vi "FPGA_DAC_buses_v2.vi"() -> ()   [LabVIEW 2013]
uses:
  <vilib>/rvi/Emulation/niFpgaSctlEmulationGetInTimedLoop.vi
  <vilib>/rvi/Memory/Memory_Emulation/niFpgaMemoryEmulationReadFromVariant.vi
  <vilib>/rvi/Memory/Memory_Emulation/niFpgaMemoryEmulationWriteToVariant.vi
  <vilib>/rvi/DataTransferAndStorage/Container/Common/niFpgaContainerGetUniqueNameForEmu.vi
  <vilib>/rvi/FIFO/Fifo_Resource/nirvififoEmulationSetSize.vi
  <vilib>/rvi/errors/niFpgaSetErrorForExecOnDevCompSimple.vi
  <vilib>/rvi/eio/common/nirviEmuReportErrorAndStop.vi
  <vilib>/rvi/Emulation/niFpgaSctlEmulationFifoFullMgr.vi
  <vilib>/rvi/Emulation/niFpgaSctlEmulationResourceMgr.vi
  <vilib>/rvi/Memory/Memory_Emulation/nirvimemoryFastEmulation.vi
  <vilib>/rvi/Memory/Memory_Emulation/nirvimemoryEmulation.vi
  <vilib>/rvi/DataTransferAndStorage/Container/XNode/niFpgaContainer.xnode
  <vilib>/rvi/FIFO/Fifo_Resource/nirvififoEmulationWrite.vi
  <vilib>/rvi/FIFO/Fifo_Resource/nirvififoEmulationRead.vi
panel:
  in  "wait(us)":u16
  in  "start movement":bool
  in  "buses to use":bool[](array[boolean])=[FALSE, FALSE, FALSE, FALSE, FALSE, FALSE, FALSE, FALSE]
  in  "stop moving bus":bool
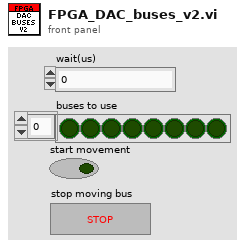
[diagram p1: front panel]
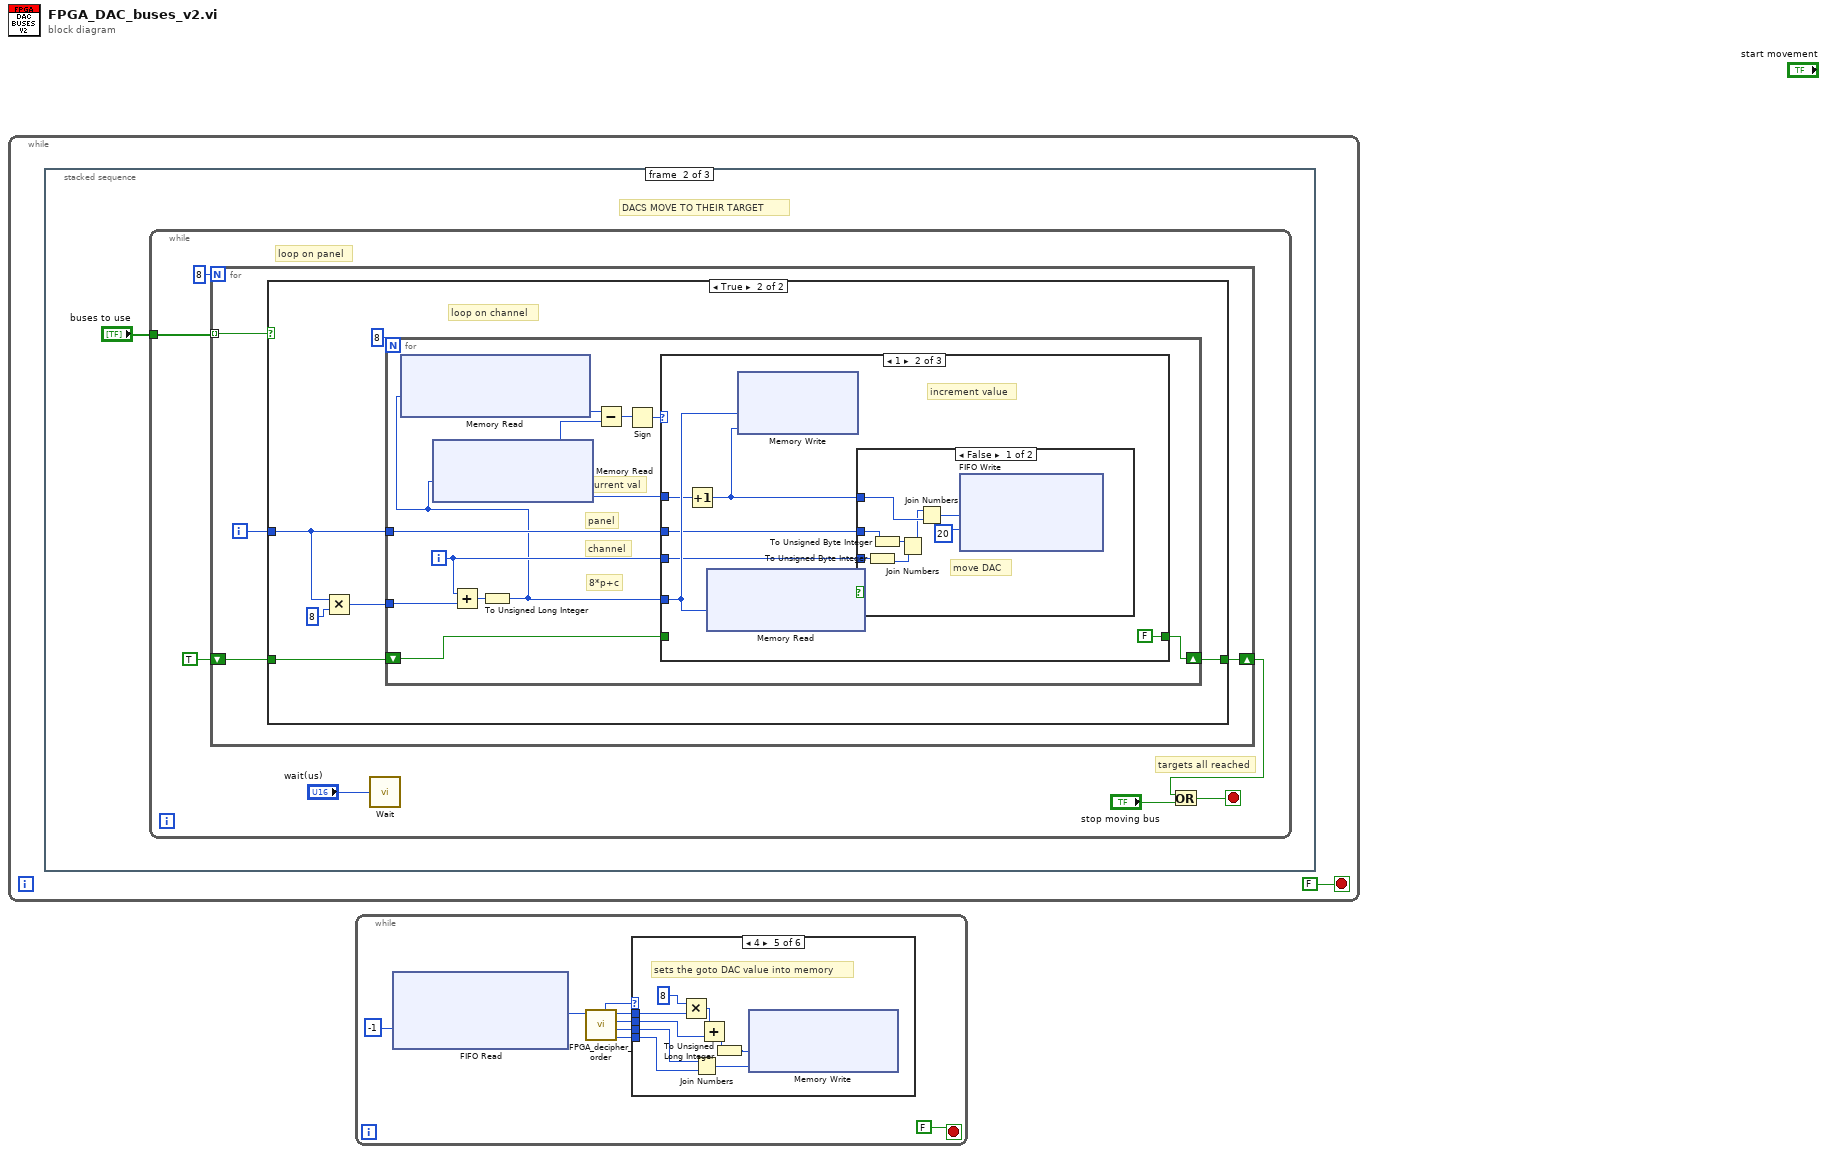
[diagram p0: block diagram]
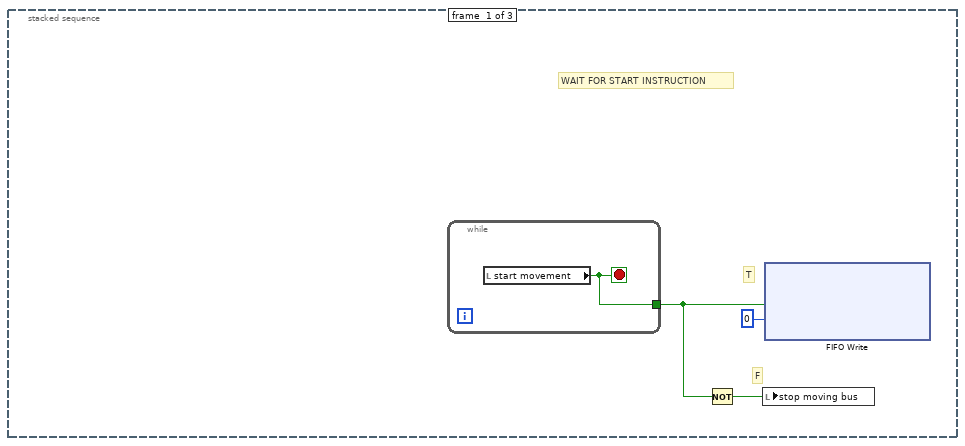
[diagram p2: hidden frame]
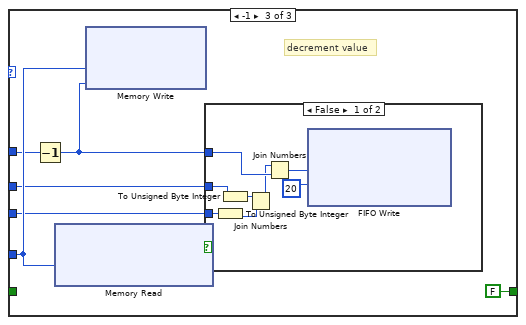
[diagram p6: hidden frame]
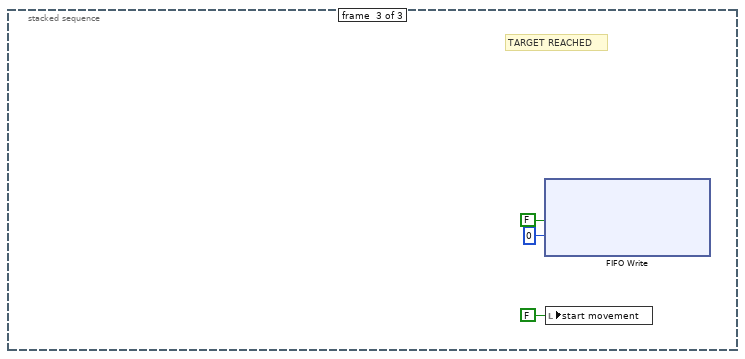
[diagram p8: hidden frame]
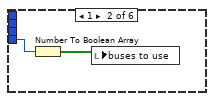
[diagram p10: hidden frame]
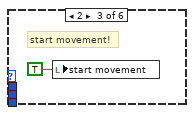
[diagram p11: hidden frame]
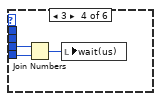
[diagram p12: hidden frame]
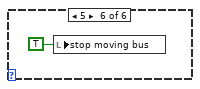
[diagram p13: hidden frame]
diagram:
  n1 = while {
    stop <- FALSE stop-if-true
    n2 = stacked-sequence {
      frame #0 {
        # "WAIT FOR START INSTRUCTION"
        # "T"
        # "F"
        n3 = while {
          tunnel: [w5] -> w3
          stop <- w5 stop-if-true
          n4 = local read "start movement"() -> (w5:bool)
        }
        n5 = Not(x=w3) -> (.not. x?=w2:bool)
        n6 = local write "stop moving bus"(w2) -> ()
        n7 = xnode ("FIFO Write")("Element"=w3, "Timeout"=0) -> ()  [unwired: 1 in, 2 out]
      }
      frame #1 {
        # "DACS MOVE TO THEIR TARGET"
        n8 = while {
          tunnel: "buses to use" -> [w8]
          stop <- w7 stop-if-true
          # "targets all reached"
          # "loop on panel"
          n9 = for {
            N: 8 -> [_]
            shift-right: [w16] -> w10
            shift-left: TRUE -> [w17]
            tunnel: w8 -> [w14] mode=indexing
            i -> [w15]
            n10 = case shown="True" w14 {
              tunnel: w15 -> [_ w21]
              tunnel: w17 -> [w18 w20]
              tunnel: [w18 w19] -> w16
              frame False {
                # "bus isn't used\nconsidered as all gates gone to value"
              }
              frame True {
                # "loop on channel"
                n11 = Multiply(x=w21, y=8) -> (x*y=w23:i32)
                n12 = for {
                  N: 8 -> [_]
                  tunnel: w23 -> [w31]
                  tunnel: w21 -> [w29]
                  shift-right: [w28] -> w19
                  shift-left: w20 -> [w27]
                  i -> [w30]
                  # "target"
                  # "8*p+c"
                  # "channel"
                  # "panel"
                  # "current val"
                  n13 = Add(x=w30, y=w31) -> (x+y=w34:i32)
                  n14 = To Unsigned Long Integer(number=w34) -> (unsigned 32bit integer=w25:u32)
                  n15 = xnode ("Memory Read")("Address"=w25) -> ("Data"=w26:u16)  [unwired: 1 in, 1 out]
                  n16 = xnode ("Memory Read")("Address"=w25) -> ("Data"=w32:u16)  [unwired: 1 in, 1 out]
                  n17 = Subtract(x=w26, y=w32) -> (x-y=w35:i32)
                  n18 = Sign(1:w35) -> (0:w33:i32)
                  n19 = case shown="1" w33 {
                    tunnel: w32 -> [_ w42 w57]
                    tunnel: w25 -> [_ w43 w58]
                    tunnel: w30 -> [_ w38 w53]
                    tunnel: w29 -> [_ w39 w54]
                    tunnel: w27 -> [w36 _ _]
                    tunnel: [w36 FALSE FALSE] -> w28
                    frame 0, Default {
                      # "target reached"
                    }
                    frame 1 {
                      # "increment value"
                      n20 = Increment(x=w42) -> (x+1=w40:u16)
                      n21 = xnode ("Memory Read")("Address"=w43) -> ("Data"=w41:bool)  [unwired: 1 in, 1 out]
                      n22 = xnode ("Memory Write")("Address"=w43, "Data"=w40) -> ()  [unwired: 1 in, 1 out]
                      n23 = case shown="False" w41 {
                        tunnel: w40 -> [w49 _]
                        tunnel: w39 -> [w48 _]
                        tunnel: w38 -> [w47 _]
                        frame False {
                          # "move DAC"
                          n24 = To Unsigned Byte Integer(number=w47) -> (unsigned 8bit integer=w46:u8)
                          n25 = To Unsigned Byte Integer(number=w48) -> (unsigned 8bit integer=w45:u8)
                          n26 = Join Numbers(hi=w45, lo=w46) -> ((hi.lo)=w44:u16)
                          n27 = Join Numbers(hi=w44, lo=w49) -> ((hi.lo)=w50:u32)
                          n28 = xnode ("FIFO Write")("Element"=w50, "Timeout"=20) -> ()  [unwired: 1 in, 2 out]
                        }
                        frame True {
                          # "DAC is used by another VI"
                        }
                      }
                    }
                    frame -1 {
                      # "decrement value"
                      n29 = Decrement(x=w57) -> (x-1=w55:u16)
                      n30 = xnode ("Memory Read")("Address"=w58) -> ("Data"=w56:bool)  [unwired: 1 in, 1 out]
                      n31 = xnode ("Memory Write")("Address"=w58, "Data"=w55) -> ()  [unwired: 1 in, 1 out]
                      n32 = case shown="False" w56 {
                        tunnel: w55 -> [w64 _]
                        tunnel: w54 -> [w63 _]
                        tunnel: w53 -> [w62 _]
                        frame False {
                          n33 = To Unsigned Byte Integer(number=w62) -> (unsigned 8bit integer=w61:u8)
                          n34 = To Unsigned Byte Integer(number=w63) -> (unsigned 8bit integer=w60:u8)
                          n35 = Join Numbers(hi=w60, lo=w61) -> ((hi.lo)=w59:u16)
                          n36 = Join Numbers(hi=w59, lo=w64) -> ((hi.lo)=w65:u32)
                          n37 = xnode ("FIFO Write")("Element"=w65, "Timeout"=20) -> ()  [unwired: 1 in, 2 out]
                        }
                        frame True {
                        }
                      }
                    }
                  }
                }
              }
            }
          }
          n38 = call "Wait"("Count(uSec)"="wait(us)") -> ()  [unwired: 1 out]
          n39 = Or(x=w10, y="stop moving bus") -> (x .or. y?=w7:bool)
        }
      }
      frame #2 {
        # "TARGET REACHED"
        n40 = xnode ("FIFO Write")("Element"=FALSE, "Timeout"=0) -> ()  [unwired: 1 in, 2 out]
        n41 = local write "start movement"(FALSE ("start movement")) -> ()
      }
    }
  }
  n42 = while {
    stop <- FALSE stop-if-true
    n43 = xnode ("FIFO Read")("Timeout"=-1) -> ("Element"=w77:u64)  [unwired: 1 in, 2 out]
    n44 = call "FPGA_decipher_order.vi"("order in"=w77) -> ("data 1"=w73:u8, "data 2"=w70:u8, "data 3"=w72:u8, "data 4"=w71:u8, "order out"=w74:u8)  [unwired: 6 out]
    n45 = case shown="4" w74 {
      tunnel: w73 -> [_ w79 _ w81 w91 _]
      tunnel: w72 -> [_ _ _ _ w85 _]
      tunnel: w71 -> [_ _ _ _ w89 _]
      tunnel: w70 -> [_ _ _ w82 w90 _]
      frame 0, Default {
      }
      frame 1 {
        n46 = Number To Boolean Array(number=w79) -> (Boolean array=w78:bool[])
        n47 = local write "buses to use"(w78) -> ()
      }
      frame 2 {
        # "start movement!"
        n48 = local write "start movement"(TRUE ("start movement")) -> ()
      }
      frame 3 {
        n49 = Join Numbers(hi=w82, lo=w81) -> ((hi.lo)=w83:u16)
        n50 = local write "wait(us)"(w83) -> ()
      }
      frame 4 {
        # "sets the goto DAC value into memory"
        n51 = Multiply(x=u8 8, y=w89) -> (x*y=w86:u8)
        n52 = Join Numbers(hi=w90, lo=w91) -> ((hi.lo)=w92:u16)
        n53 = Add(x=w86, y=w85) -> (x+y=w87:u8)
        n54 = To Unsigned Long Integer(number=w87) -> (unsigned 32bit integer=w84:u32)
        n55 = xnode ("Memory Write")("Address"=w84, "Data"=w92) -> ()  [unwired: 1 in, 1 out]
      }
      frame 5 {
        n56 = local write "stop moving bus"(TRUE ("stop moving bus")) -> ()
      }
    }
  }
